vi "Future Usage - Timeouts.vi"   [LabVIEW 2017]
uses:
  <vilib>/Utility/error.llb/Error Cluster From Error Code.vi
  <vilib>/ErrorRing/Error Ring.xnode
  Futures/Futures.lvlib
  Futures/Future/Future.lvclass
  Futures/Promise/Promise.lvclass
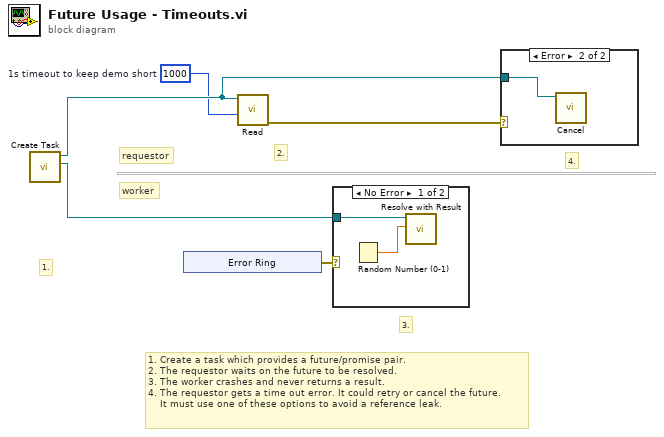
[diagram p0: block diagram]
diagram:
  w1 = 1000  # 1s timeout to keep demo short
  # "3."
  # "4."
  # "2."
  # "1. Create a task which provides a future/promise pair.\n2. The requestor waits on the future to be resolved.\n3. The worker crashes and never returns a result.\n4. The requestor gets a time out error. It could retry or cancel the future. \n    It must use one of these options to avoid a reference leak."
  # "requestor"
  # "worker"
  # "1."
  n1 = call "Create Task.vi"() -> ("Promise out"=w5:refnum<class "Promise.lvclass">, "Future out"=w2:refnum<class "Future.lvclass">)  [unwired: 9 in, 1 out]
  n2 = xnode "Error Ring"() -> ("error out"=w4:errorcluster)
  n3 = call "Read.vi"("timeout in ms (60 sec)"=w1, "Future in"=w2) -> ("error out"=w3:errorcluster)  [unwired: 6 in, 3 out]
  n4 = case shown="No Error" w4 {
    tunnel: w5 -> [w7 _]
    frame No Error {
      n5 = Random Number (0-1)() -> (number: 0 to 1=w6:dbl)
      n6 = call "Resolve with Result.vi"("Result"=w6, "Promise in"=w7) -> ()  [unwired: 9 in, 1 out]
    }
    frame Error {
    }
  }
  n7 = case shown="Error" w3 {
    tunnel: w2 -> [_ w8]
    frame No Error {
    }
    frame Error {
      n8 = call "Cancel.vi"("Future in"=w8) -> ()  [unwired: 10 in, 1 out]
    }
  }
